vi "Section off entire jump.vi"(6 "System Weight":dbl, 7 "Jump Edge Detection\nThreshold (Default is 5)":dbl, 8 "Force Plate Ringing\nOffset Length":dbl, 9 "Dynamic Data Type":dynamicdata(waveform), 10 "Beginning Cursor":dbl, 11 "Ending Cursor":dbl) -> (0 "Jump Offset from V=0":i32, 1 "Entire Jump Starting at V=0":dbl[](array[numeric]), 2 "Flight Time Array":dbl[](array[numeric]), 3 "Entire Jump Array":dbl[](array[numeric]), 4 "Section Between Cursors":dbl[](array[numeric]))   [LabVIEW 2016]
uses:
  <vilib>/measure/mamon.llb/Trigger Detection for 1 Channel.vi
  <vilib>/measure/NI_MAPro.lvlib
panel:
  out "Section":dynamicdata(graph)
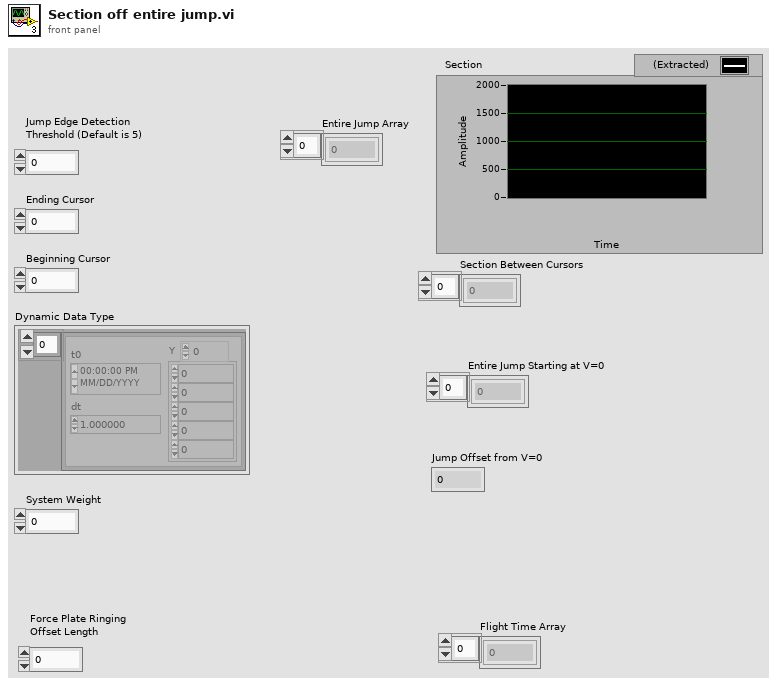
[diagram p1: front panel]
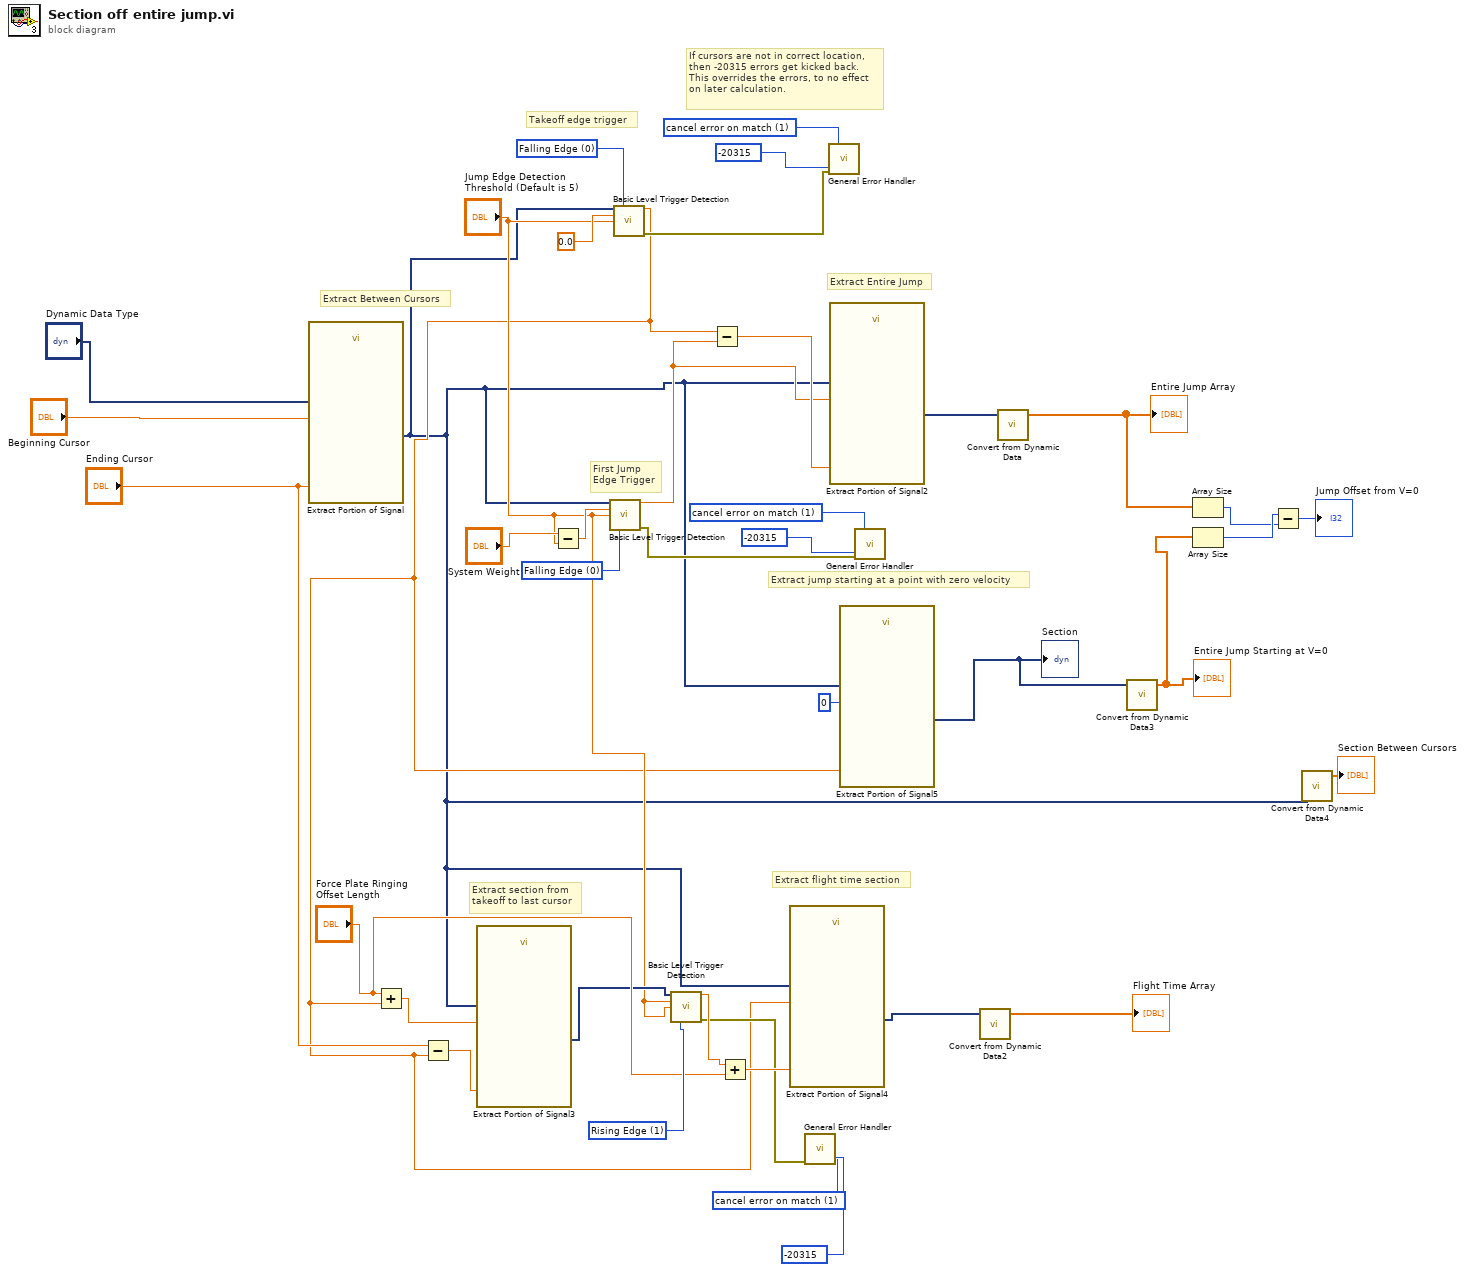
[diagram p0: block diagram]
diagram:
  w12 = 1 items=["no exception", "cancel error on match", "set error on match"] ("[exception action] (none:0)")
  w14 = 1 items=["no exception", "cancel error on match", "set error on match"] ("[exception action] (none:0)")
  w17 = 1 items=["no exception", "cancel error on match", "set error on match"] ("[exception action] (none:0)")
  w31 = u16 1 items=["Falling Edge", "Rising Edge"] ("trigger slope")
  w40 = u16 0 items=["Falling Edge", "Rising Edge"] ("trigger slope")
  w37 = u16 0 items=["Falling Edge", "Rising Edge"] ("trigger slope")
  # "Extract jump starting at a point with zero velocity"
  # "If cursors are not in correct location,\nthen -20315 errors get kicked back. \nThis overrides the errors, to no effect\non later calculation."
  # "Extract flight time section"
  # "Extract section from\ntakeoff to last cursor"
  # "Takeoff edge trigger"
  # "First Jump \nEdge Trigger"
  # "Extract Entire Jump"
  # "Extract Between Cursors"
  n1 = call "Extract Portion of Signal"("Samples"="Ending Cursor", "Begin Sample"="Beginning Cursor", "Signals"="Dynamic Data Type") -> ("Section"=w2:dynamicdata)  [unwired: 7 in, 1 out]
  n2 = Subtract(x="System Weight", y="Jump Edge Detection\nThreshold (Default is 5)") -> (x-y=w22:dbl)
  n3 = call-poly <vilib>:"Basic Level Trigger Detection.vi"("signal in"=w2, "level"=w22, "hysteresis"="Jump Edge Detection\nThreshold (Default is 5)", "trigger slope"=w40) -> ("trigger location"=w34:dbl, "error out"=w15:errorcluster)  [unwired: 9 in, 1 out]
  n4 = call-poly <vilib>:"Basic Level Trigger Detection.vi"("signal in"=w2, "level"=0.0, "hysteresis"="Jump Edge Detection\nThreshold (Default is 5)", "trigger slope"=w37) -> ("trigger location"=w9:dbl, "error out"=w11:errorcluster)  [unwired: 9 in, 1 out]
  n5 = Add(x="Force Plate Ringing\nOffset Length", y=w9) -> (x+y=w28:dbl)
  n6 = Subtract(x="Ending Cursor", y=w9) -> (x-y=w32:dbl)
  n7 = call "Extract Portion of Signal3"("Samples"=w32, "Begin Sample"=w28, "Signals"=w2) -> ("Section"=w24:dynamicdata)  [unwired: 7 in, 1 out]
  n8 = call-poly <vilib>:"Basic Level Trigger Detection.vi"("signal in"=w24, "level"="Jump Edge Detection\nThreshold (Default is 5)", "hysteresis"="Jump Edge Detection\nThreshold (Default is 5)", "trigger slope"=w31) -> ("trigger location"=w26:dbl, "error out"=w19:errorcluster)  [unwired: 9 in, 1 out]
  n9 = Subtract(x=w9, y=w34) -> (x-y=w38:dbl)
  n10 = Add(x=w26, y="Force Plate Ringing\nOffset Length") -> (x+y=w27:dbl)
  n11 = call "Extract Portion of Signal4"("Samples"=w27, "Begin Sample"=w9, "Signals"=w2) -> ("Section"=w29:dynamicdata)  [unwired: 7 in, 1 out]
  n12 = call <vilib>:"General Error Handler.vi"("error in (no error)"=w19, "[exception action] (none:0)"=w17, "[exception code]"=-20315 ("error code (no error:0)")) -> ()  [unwired: 8 in, 5 out]
  n13 = call <vilib>:"General Error Handler.vi"("error in (no error)"=w11, "[exception action] (none:0)"=w12, "[exception code]"=-20315 ("error code (no error:0)")) -> ()  [unwired: 8 in, 5 out]
  n14 = call "Extract Portion of Signal2"("Samples"=w38, "Begin Sample"=w34, "Signals"=w2) -> ("Section"=w39:dynamicdata)  [unwired: 7 in, 1 out]
  n15 = call "Extract Portion of Signal5"("Samples"=w9, "Begin Sample"=0, "Signals"=w2) -> ("Section"=w8:dynamicdata)  [unwired: 7 in, 1 out]
  "Section" <- w8
  n16 = call <vilib>:"General Error Handler.vi"("error in (no error)"=w15, "[exception action] (none:0)"=w14, "[exception code]"=-20315 ("error code (no error:0)")) -> ()  [unwired: 8 in, 5 out]
  n17 = call "Convert from Dynamic Data2"("Dynamic Data Type"=w29) -> ("Array"=→"Flight Time Array":dbl[])  [unwired: 3 in]
  n18 = call "Convert from Dynamic Data"("Dynamic Data Type"=w39) -> ("Array"=w7:dbl[])  [unwired: 3 in]
  "Entire Jump Array" <- w7
  n19 = call "Convert from Dynamic Data3"("Dynamic Data Type"=w8) -> ("Array"=w6:dbl[])  [unwired: 3 in]
  "Entire Jump Starting at V=0" <- w6
  n20 = Array Size(array=w7) -> (size(s)=w4:i32)
  n21 = Array Size(array=w6) -> (size(s)=w5:i32)
  n22 = Subtract(x=w5, y=w4) -> (x-y=→"Jump Offset from V=0":i32)
  n23 = call "Convert from Dynamic Data4"("Dynamic Data Type"=w2) -> ("Array"=→"Section Between Cursors":dbl[])  [unwired: 3 in]
